vi "DBToString.vi"(8 "Enum":T1=enum."UseLauncherPID") -> (1 "Refname":string)   [LabVIEW 2012]
uses:
  Sally_Dashboard_2013/DBNameEnum.ctl
panel:
  in  "RefnameArray":string[](array[string])=["AutoEnum", "DriveLoopTime", "DriveAlignLS", "ClimbLS", "LauncherAngleMatches", "FrameworkVision", "sLauncherAngle", "LauncherTargetAngle", "sLauncherRPM", "LauncherTargetRPM", "sDriveDistance", "LauncherMotorValue", "PullbackTol", "FireTol", "LauncherRPMTol", "LauncherAngleTol", "BackRight", "CloseLeft", "BehindPyramid", "Disabled", "CloseRight", "BackLeft", "InitialWait", "WaitBetweenLaunch", "AngleCluster", "RPMCluster", "UseAngleEncoder", "UseLauncherEncoder", "UseLauncherPID"]
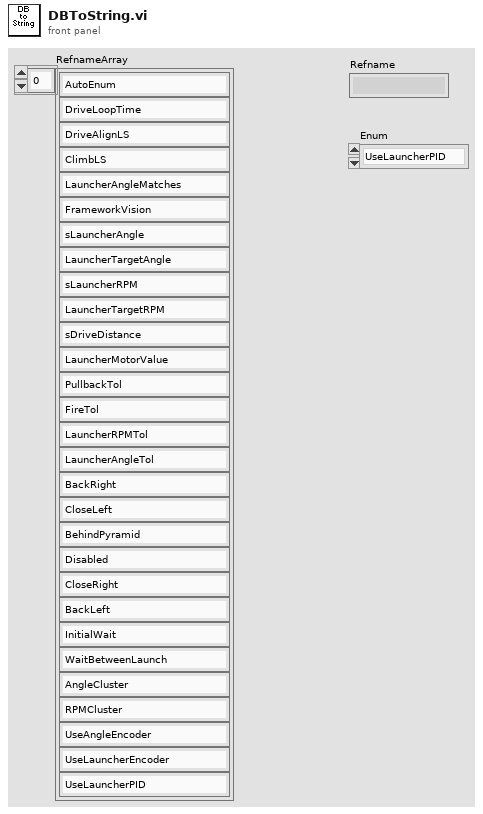
[diagram p1: front panel]
types:
  T1 = typedef "DBNameEnum.ctl" = enum16{"AutoEnum", "DriveLoopTime", "DriveAlignLS", "ClimbLS", "LauncherAngleMatches", "FrameworkVersion", "sLauncherAngle", "LauncherTargetAngle", "sLauncherRPM", "LauncherTargetRPM", "sDriveDistance", "LauncherMotorValue", "PullbackTol", "FireTol", "LauncherRPMTol", "LauncherAngleTol", "BackRight", "CloseLeft", "BehindPyramid", "Disabled", "CloseRight", "BackLeft", "InitialWait", "WaitBetweenLaunch", "AngleCluster", "RPMCluster", "UseAngleEncoder", "UseLauncherEncoder", "UseLauncherPID"}
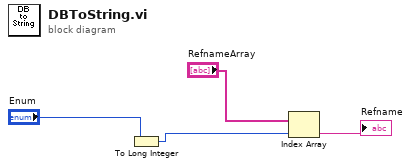
[diagram p0: block diagram]
diagram:
  n1 = To Long Integer(number="Enum") -> (32bit integer=w2:i32)
  n2 = Index Array(array="RefnameArray", index=w2) -> (element=→"Refname":string)
